vi "Apply Item Name to Ring.vi"(8 "error in":errorcluster, 10 "Item Name":string, 11 "Ring in":refnum<vi>) -> (0 "error out":errorcluster)   [LabVIEW 2020, in "Panther Dashboard.lvlib"]
uses:
  Panther Dashboard.lvlib
  e066e9a3-9089-452e-b790-f53ff6244b07.vi
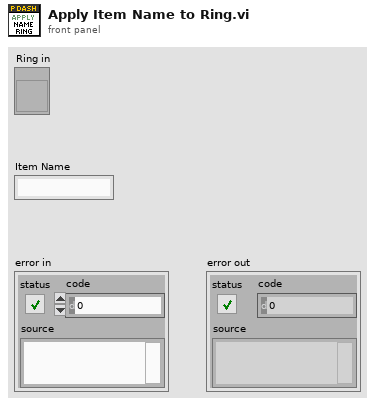
[diagram p1: front panel]
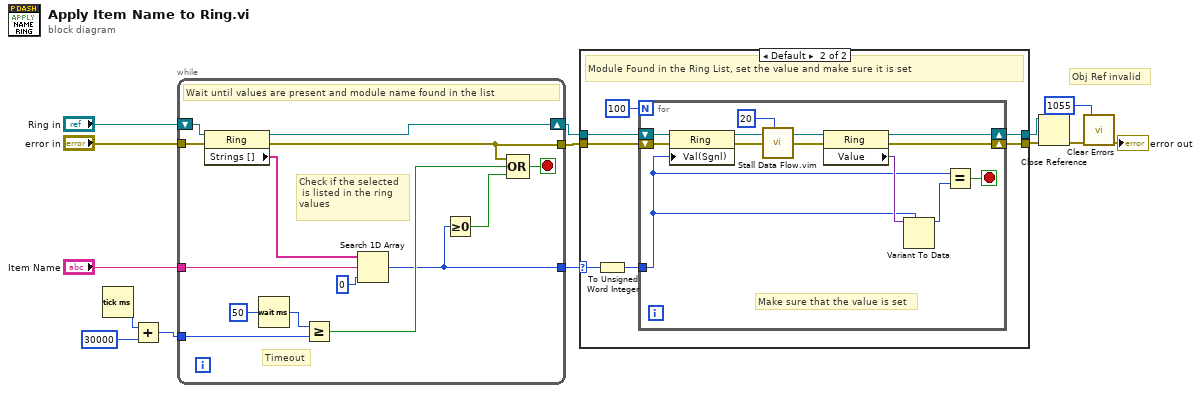
[diagram p0: block diagram]
diagram:
  # "Obj Ref invalid"
  n1 = Tick Count (ms)() -> (millisecond timer value=w6:u32)
  n2 = Add(x=w6, y=u32 30000) -> (x+y=w10:u32)
  n3 = while {
    shift-right: [w26] -> w4
    shift-left: "Ring in" -> [w25]
    tunnel: "error in" -> [w28]
    tunnel: [w27] -> w11
    tunnel: w10 -> [w20]
    tunnel: [w16] -> w7
    tunnel: "Item Name" -> [w15]
    stop <- w23 stop-if-true
    # "Timeout"
    # "Check if the selected\n is listed in the ring\nvalues"
    # "Wait until values are present and module name found in the list"
    n4 = property class="Ring"(reference=w25, error in=w28) -> (reference out=w26:refnum<vi>, error out=w27:errorcluster, "Strings []"=w18:string[])
    n5 = Wait (ms)(milliseconds to wait=u32 50) -> (millisecond timer value=w22:u32)
    n6 = Greater Or Equal?(x=w22, y=w20) -> (x >= y?=w24:bool)
    n7 = Search 1D Array(1D array=w18, element=w15, start index (0)=0) -> (index of element=w16:i32)
    n8 = Greater Or Equal To 0?(x=w16) -> (x >= 0?=w17:bool)
    n9 = Compound Arithmetic op=OR(w27, w24, w17) -> (w23:bool)
  }
  n10 = case shown="Default" w7 {
    selector: w7 -> [_ w35]
    tunnel: w4 -> [w29 w34]
    tunnel: [w29 w32] -> w8
    tunnel: w11 -> [w30 w37]
    tunnel: [w30 w36] -> w12
    frame -1 {
      # "Module name not found in the ring list"
    }
    frame Default {
      # "Module Found in the Ring List, set the value and make sure it is set"
      n11 = To Unsigned Word Integer(number=w35) -> (unsigned 16bit integer=w33:u16)
      n12 = for {
        N: 100 -> [_]
        tunnel: w33 -> [w40]
        shift-right: [w47] -> w36
        shift-left: w37 -> [w49]
        shift-right: [w43] -> w32
        shift-left: w34 -> [w45]
        stop <- w39 stop-if-true
        # "Make sure that the value is set"
        n13 = property class="Ring"(reference=w45, error in=w49, "Val(Sgnl)"=w40) -> (reference out=w44:refnum<vi>, error out=w48:errorcluster)
        n14 = call "Stall Data Flow.vim"("value in"=w48, "milliseconds to wait"=u32 20) -> ("value out"=w46:errorcluster)  [unwired: 1 out]
        n15 = property class="Ring"(reference=w44, error in=w46) -> (reference out=w43:refnum<vi>, error out=w47:errorcluster, "Value"=w42:variant)
        n16 = Variant To Data(type=w40, Variant=w42) -> (data=w41:u16)  [unwired: 1 in, 1 out]
        n17 = Equal?(x=w40, y=w41) -> (x = y?=w39:bool)
      }
    }
  }
  n18 = Close Reference(reference=w8, error in (no error)=w12) -> (error out=w13:errorcluster)
  n19 = call <vilib>:"Clear Errors.vi"("error in (no error)"=w13, "specific error code to clear (0: all)"=1055) -> ("error out"=→"error out":errorcluster)  [unwired: 4 in, 1 out]
